vi "Vending Machine PC.vi"() -> ()   [LabVIEW 2019]
doc: "Use this template to build a producer/consumer design pattern with events to produce queue items. Use this design pattern instead of the User Interface Event Handler pattern for user interfaces when you want to execute code asynchronously in response to an event without slowing the user interface responsiveness."
uses:
  Controls/States.ctl
panel:
  in  "Path":path=path "C:/Users/user/Google 드라이브/Jeonghwa/Labview/Labiview 2018/Vending Machine (Exam)/Configuration Data File.ini"
  out "error out":errorcluster={"status"=TRUE, "code"=7, "source"="Open/Create/Replace File in NI_LVConfig.lvlib:Load.vi->NI_LVConfig.lvlib:Open Config Data.vi->Configuration.vi->Vending Machine main.vi<APPEND>\nC:\\Users\\user\\Google 드라이브\\Jeonghwa\\Labview\\Labiview 2018\\Exam\\Configuration Data File.ini"}
  in  "Stop Button":bool
  out "Elapsed time":dbl format="%#.2g"
  out "Dispatch":bool
  in  "Selector":T1
  out "Row":i32
  in  "Deposit":bool
  in  "Return":bool
  in  "Menus":T2(array[cluster])
  out "Amount ($)":dbl
  out "Change":dbl
  in  "error in":errorcluster
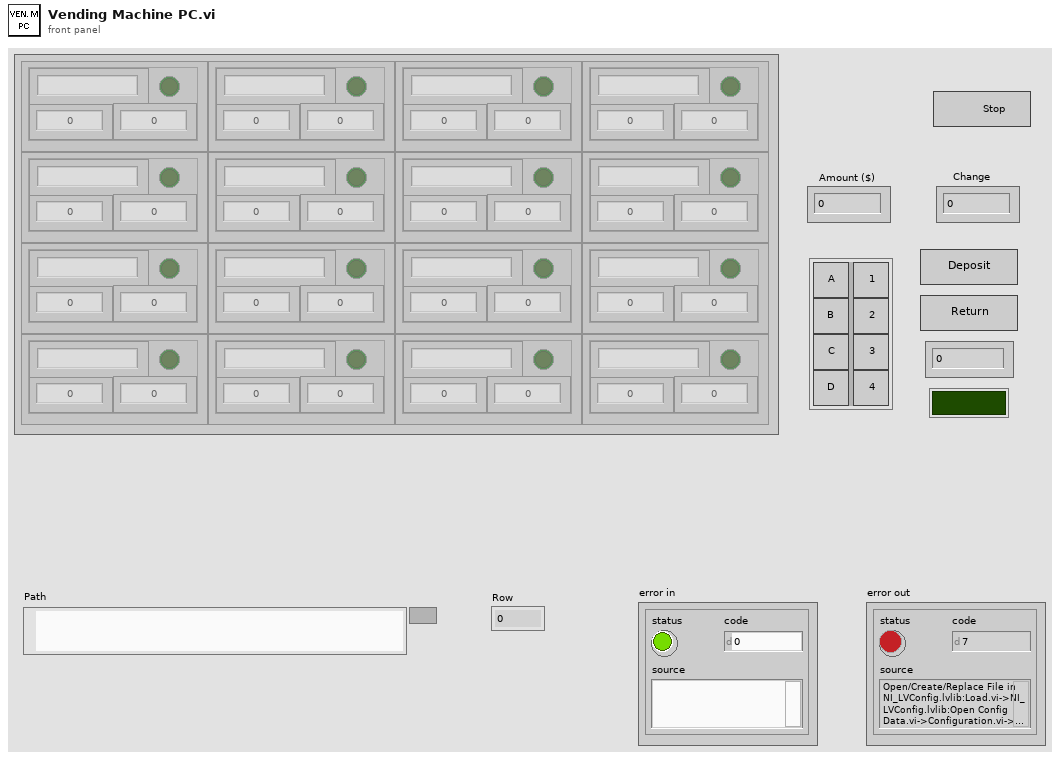
[diagram p1: front panel]
types:
  T1 = cluster{"A":bool, "B":bool, "C":bool, "D":bool, "1":bool, "2":bool, "3":bool, "4":bool}
  T2 = cluster{"Price":dbl, "Name":string, "Left":u32, "Available":bool}[][]
  T3 = typedef "States.ctl" = enum16{"Initial", "Dispatch", "Stop"}
  T4 = cluster{"Price":dbl, "Name":string, "Left":u32, "Available":bool}
  T5 = cluster{"Price":u32, "Name":string, "Left":u32, "Available":bool}[][]
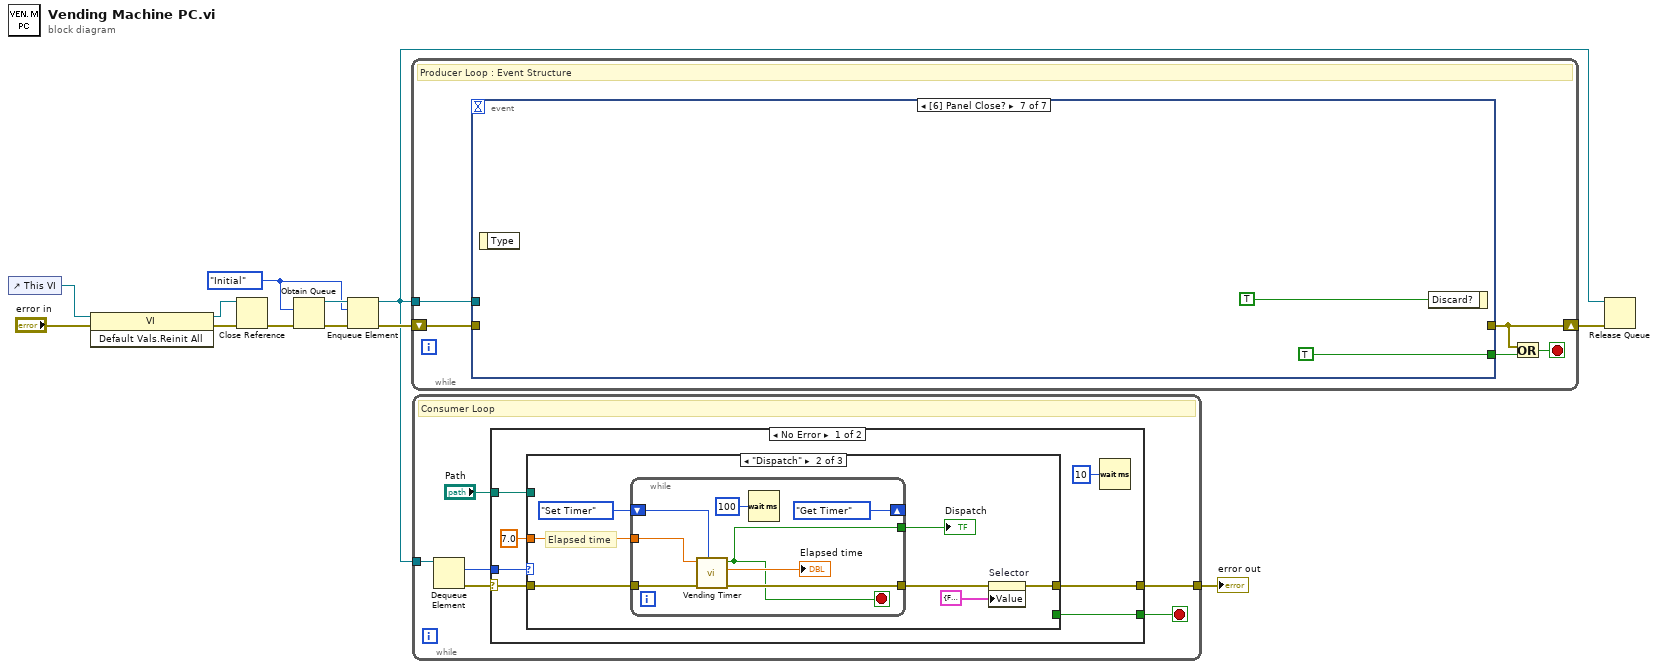
[diagram p0: block diagram]
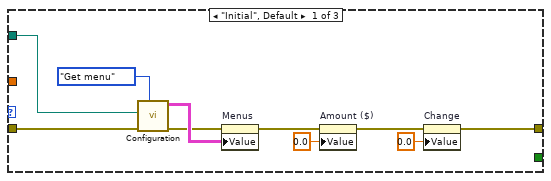
[diagram p2: hidden frame]
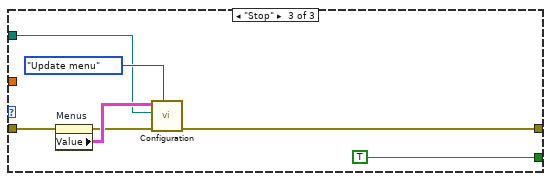
[diagram p3: hidden frame]
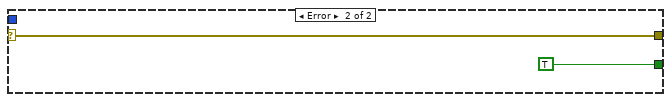
[diagram p4: hidden frame]
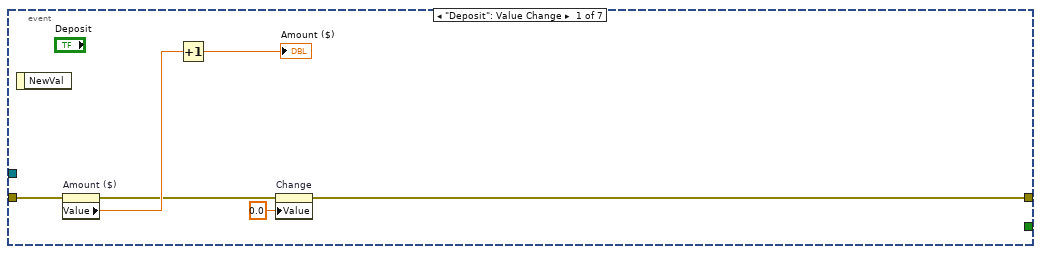
[diagram p5: hidden frame]
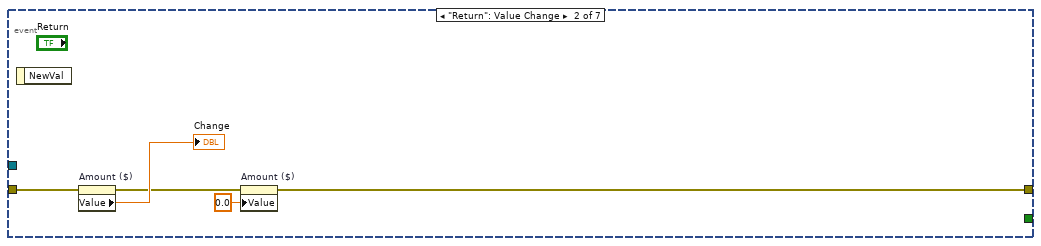
[diagram p6: hidden frame]
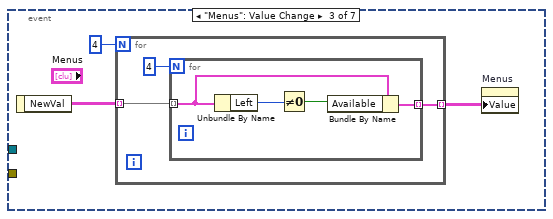
[diagram p7: hidden frame]
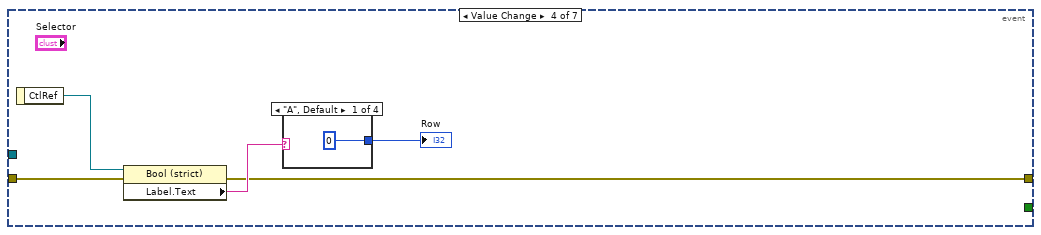
[diagram p8: hidden frame]
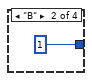
[diagram p9: hidden frame]
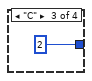
[diagram p10: hidden frame]
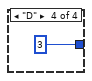
[diagram p11: hidden frame]
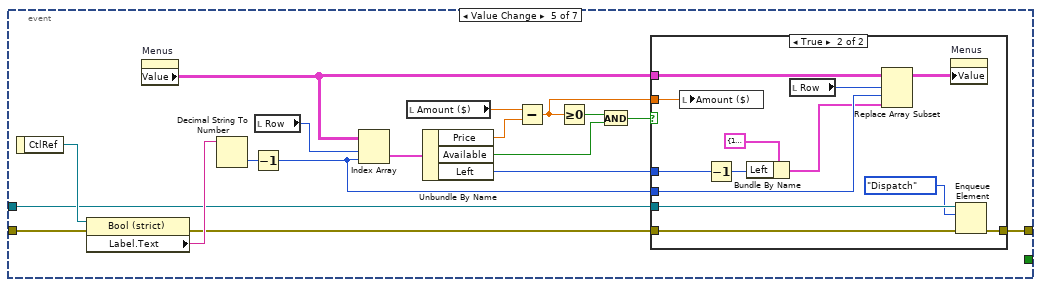
[diagram p12: hidden frame]
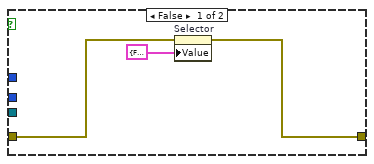
[diagram p13: hidden frame]
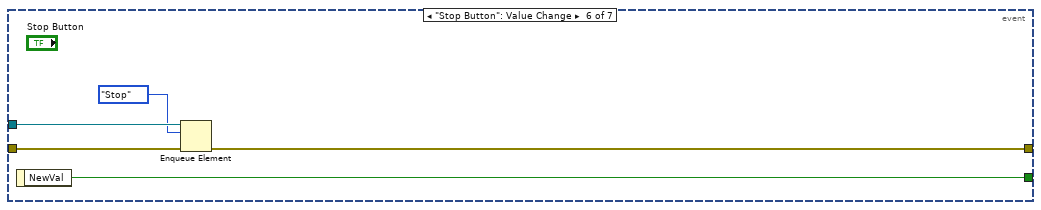
[diagram p14: hidden frame]
diagram:
  w7 = States."Initial" ("States")
  n1 = control-ref of="This VI"() -> (w6:refnum<vi>)
  n2 = invoke class="VI" method="Default Vals.Reinit All"(reference=w6, error in="error in") -> (reference out=w5:refnum<vi>, error out=w4:errorcluster)  [unwired: 1 in, 1 out]
  n3 = Close Reference(reference=w5, error in (no error)=w4) -> (error out=w2:errorcluster)
  n4 = Obtain Queue(element data type=w7, error in (no error)=w2) -> (queue out=w9:refnum<queue>, error out=w11:errorcluster)  [unwired: 3 in, 1 out]
  n5 = Enqueue Element(queue=w9, element=w7, error in (no error)=w11) -> (queue out=w8:refnum<queue>, error out=w10:errorcluster)  [unwired: 1 in, 1 out]
  n6 = while {
    shift-right: [w13] -> w12
    shift-left: w10 -> [w16]
    tunnel: w8 -> [w17]
    stop <- w14 stop-if-true
    # "Producer Loop : Event Structure"
    n7 = event shown="[6] Panel Close?" {
      selector: _ -> [_ _ _ _ _ _ _]
      dyn-events: _ -> [_ _ _ _ _ _ _]
      timeout: _ -> [_ _ _ _ _ _ _]
      tunnel: w17 -> [_ _ _ _ w59 w84 _]
      tunnel: w16 -> [w22 w28 _ w42 w64 w85 _]
      tunnel: [w18 w24 _ w40 w58 w82 _] -> w13
      tunnel: [_ _ _ _ _ w86 TRUE ("NewVal")] -> w15
      event "Deposit": Value Change {
        n8 = event-data() -> ()  [unwired: 1 in, 1 out]
        n9 = property on="Amount ($)" class="DigNum (strict)"(error in=w22) -> (error out=w19:errorcluster, "Value"=w23:dbl)  [unwired: 1 in, 1 out]
        n10 = Increment(x=w23) -> (x+1=→"Amount ($)":dbl)
        n11 = property on="Change" class="DigNum (strict)"(error in=w19, "Value"=0.0 ("Change")) -> (error out=w18:errorcluster)  [unwired: 1 in, 1 out]
      }
      event "Return": Value Change {
        n12 = event-data() -> ()  [unwired: 1 in, 1 out]
        n13 = property on="Amount ($)" class="DigNum (strict)"(error in=w28) -> (error out=w25:errorcluster, "Value"=→"Change":dbl)  [unwired: 1 in, 1 out]
        n14 = property on="Amount ($)" class="DigNum (strict)"(error in=w25, "Value"=0.0 ("Amount ($)")) -> (error out=w24:errorcluster)  [unwired: 1 in, 1 out]
      }
      event "Menus": Value Change {
        n15 = event-data() -> ("NewVal"=w29:T2)  [unwired: 1 in]
        n16 = for {
          N: 4 -> [_]
          tunnel: w29 -> [w33] mode=indexing
          tunnel: [w32] -> w30 mode=indexing
          n17 = for {
            N: 4 -> [_]
            tunnel: w33 -> [w35] mode=indexing
            tunnel: [w36] -> w32 mode=indexing
            n18 = Unbundle By Name(w35) -> ("Left"=w37:u32)
            n19 = Not Equal To 0?(x=w37) -> (x != 0?=w38:bool)
            n20 = Bundle By Name(cluster=w35, "Available"=w38) -> (w36:T4)
          }
        }
        n21 = property on="Menus" class="Arr (strict)"("Value"=w30) -> ()  [unwired: 2 in, 2 out]
      }
      event "Selector.A", "Selector.B", "Selector.C", "Selector.D": Value Change {
        n22 = event-data() -> ("CtlRef"=w41:refnum<vi>)  [unwired: 1 in]
        n23 = property class="Bool (strict)"(reference=w41, error in=w42) -> (error out=w40:errorcluster, "Label.Text"=w43:string)  [unwired: 1 out]
        n24 = case shown="\"A\", Default" w43 {
          tunnel: [0 1 2 3] -> w39
          frame "A", Default {
          }
          frame "B" {
          }
          frame "C" {
          }
          frame "D" {
          }
        }
        "Row" <- w39
      }
      event "Selector.1", "Selector.2", "Selector.3", "Selector.4": Value Change {
        n25 = event-data() -> ("CtlRef"=w65:refnum<vi>)  [unwired: 1 in]
        n26 = property class="Bool (strict)"(reference=w65, error in=w64) -> (error out=w51:errorcluster, "Label.Text"=w63:string)  [unwired: 1 out]
        n27 = property on="Menus" class="Arr (strict)"() -> ("Value"=w50:T2)  [unwired: 2 in, 2 out]
        n28 = Decimal String To Number(string=w63) -> (number=w49:i32)  [unwired: 2 in, 1 out]
        n29 = Decrement(x=w49) -> (x-1=w48:i32)
        n30 = local read "Row"() -> (w62:i32)
        n31 = Index Array(array=w50, index (row)=w62, index (col)=w48) -> (element=w61:T4)
        n32 = local read "Amount ($)"() -> (w53:dbl)
        n33 = Unbundle By Name(w61) -> ("Price"=w55:dbl, "Available"=w60:bool, "Left"=w56:u32)
        n34 = Subtract(x=w53, y=w55) -> (x-y=w52:dbl)
        n35 = Greater Or Equal To 0?(x=w52) -> (x >= 0?=w54:bool)
        n36 = And(x=w54, y=w60) -> (x .and. y?=w57:bool)
        n37 = case shown="True" w57 {
          tunnel: w59 -> [_ w81]
          tunnel: w51 -> [w67 w80]
          tunnel: [w66 w78] -> w58
          tunnel: w56 -> [_ w76]
          tunnel: w52 -> [_ w69]
          tunnel: w50 -> [_ w75]
          tunnel: w48 -> [_ w73]
          frame False {
            n38 = property on="Selector" class="Clust (strict)"(error in=w67, "Value"=T1 {"A"=FALSE, "B"=FALSE, "C"=FALSE, "D"=FALSE, "1"=FALSE, "2"=FALSE, "3"=FALSE, "4"=FALSE} ("Selector")) -> (error out=w66:errorcluster)  [unwired: 1 in, 1 out]
          }
          frame True {
            n39 = local write "Amount ($)"(w69) -> ()
            n40 = Decrement(x=w76) -> (x-1=w77:u32)
            n41 = Bundle By Name(cluster=T4 {"Price"=1.0, "Name"="Cola1", "Left"=94, "Available"=TRUE} ("Items"), "Left"=w77) -> (w72:T4)
            n42 = local read "Row"() -> (w74:i32)
            n43 = Replace Array Subset(array=w75, new element=w72, index (row)=w74, index (col)=w73) -> (w71:T2)
            n44 = property on="Menus" class="Arr (strict)"("Value"=w71) -> ()  [unwired: 2 in, 2 out]
            n45 = Enqueue Element(queue=w81, element=States."Dispatch", error in (no error)=w80) -> (error out=w78:errorcluster)  [unwired: 1 in, 2 out]
          }
        }
      }
      event "Stop Button": Value Change {
        n46 = event-data() -> ("NewVal"=w86:bool)  [unwired: 1 in]
        n47 = Enqueue Element(queue=w84, element=States."Stop", error in (no error)=w85) -> (error out=w82:errorcluster)  [unwired: 1 in, 2 out]
      }
      event Panel Close? {
        n48 = event-data() -> ()  [unwired: 1 in, 1 out]
        n49 = event-data("Discard?"=TRUE) -> ()  [unwired: 1 in, 1 out]
      }
    }
    n50 = Or(x=w13, y=w15) -> (x .or. y?=w14:bool)
  }
  n51 = while {
    tunnel: w8 -> [w94]
    tunnel: [w89] -> w1
    stop <- w91 stop-if-true
    # "Consumer Loop"
    n52 = Dequeue Element(queue=w94) -> (element=w92:T3, error out=w93:errorcluster)  [unwired: 2 in, 2 out]
    n53 = case shown="No Error" w93 {
      selector: w93 -> [w98 w134]
      tunnel: w92 -> [w100 _]
      tunnel: [w96 TRUE] -> w91
      tunnel: "Path" -> [w99 _]
      tunnel: [w97 w134] -> w89
      frame No Error {
        n54 = case shown="\"Dispatch\"" w100 {
          tunnel: w99 -> [w109 _ w127]
          tunnel: w98 -> [w110 w117 w129]
          tunnel: [w102 w113 w128] -> w97
          tunnel: [_ _ TRUE] -> w96
          tunnel: 7.0 ("Target Time") -> [_ w116 _]
          frame "Initial", Default {
            n55 = call "Configuration.vi"("Get/Set"=enum16{"Get menu", "Update menu"}."Get menu" ("Get/Update"), "Error In"=w110, "File Path"=w109) -> ("Error Out"=w107:errorcluster, "Menus out"=w108:T5)  [unwired: 7 in]
            n56 = property on="Menus" class="Arr (strict)"(error in=w107, "Value"=w108) -> (error out=w106:errorcluster)  [unwired: 1 in, 1 out]
            n57 = property on="Amount ($)" class="DigNum (strict)"(error in=w106, "Value"=0.0 ("Amount ($)")) -> (error out=w104:errorcluster)  [unwired: 1 in, 1 out]
            n58 = property on="Change" class="DigNum (strict)"(error in=w104, "Value"=0.0 ("Change")) -> (error out=w102:errorcluster)  [unwired: 1 in, 1 out]
          }
          frame "Dispatch" {
            # "Elapsed time"
            n59 = while {
              shift-right: [enum16{"Get Timer", "Set Timer"}."Get Timer" ("Set/Get")] -> _
              shift-left: enum16{"Get Timer", "Set Timer"}."Set Timer" ("Set/Get") -> [w126]
              tunnel: w117 -> [w124]
              tunnel: w116 -> [w123]
              tunnel: [w121] -> w115
              tunnel: [w120] -> w112
              stop <- w120 stop-if-true
              n60 = call "Vending Timer.vi"("Set/Get"=w126, "Error In"=w124, "Target Time"=w123) -> ("Error Out"=w121:errorcluster, "Elapsed Time"=→"Elapsed time":dbl, "Elapsed?"=w120:bool)  [unwired: 4 in]
              n61 = Wait (ms)(milliseconds to wait=u32 100) -> ()  [unwired: 1 out]
            }
            "Dispatch" <- w112
            n62 = property on="Selector" class="Clust (strict)"(error in=w115, "Value"=T1 {"A"=FALSE, "B"=FALSE, "C"=FALSE, "D"=FALSE, "1"=FALSE, "2"=FALSE, "3"=FALSE, "4"=FALSE} ("Selector")) -> (error out=w113:errorcluster)  [unwired: 1 in, 1 out]
          }
          frame "Stop" {
            n63 = property on="Menus" class="Arr (strict)"(error in=w129) -> (error out=w130:errorcluster, "Value"=w131:T2)  [unwired: 1 in, 1 out]
            n64 = call "Configuration.vi"("Get/Set"=enum16{"Get menu", "Update menu"}."Update menu" ("Get/Update"), "Error In"=w130, "File Path"=w127, "Menus"=w131) -> ("Error Out"=w128:errorcluster)  [unwired: 6 in, 1 out]
          }
        }
        n65 = Wait (ms)(milliseconds to wait=u32 10) -> ()  [unwired: 1 out]
      }
      frame Error {
      }
    }
  }
  "error out" <- w1
  n66 = Release Queue(queue=w8, error in (no error)=w12) -> ()  [unwired: 1 in, 3 out]
